vi "Register Voter.vi"(9 "VoterInfo":cluster{"VoterName":string, "Ballot":string}, 10 "VoterID":i32, 11 "map in":T1(c390)) -> (3 "map out":T1(c390))   [LabVIEW 2019]
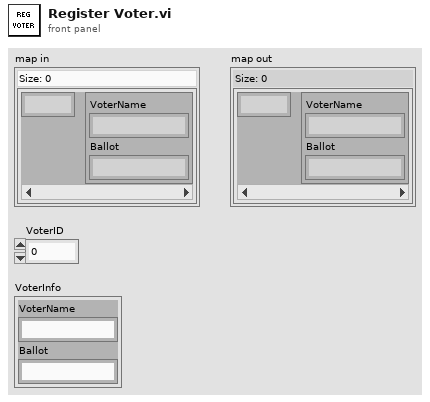
[diagram p1: front panel]
types:
  T1 = map{i32, cluster{"VoterName":string, "Ballot":string}}
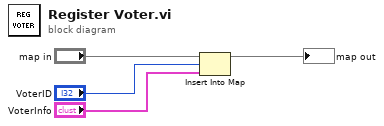
[diagram p0: block diagram]
diagram:
  n1 = Insert Into Map(map in="map in", key="VoterID", value="VoterInfo") -> (map out=→"map out":T1)  [unwired: 2 out]
